vi "Menu Launch VI Information.vi"(8 "error in (no error)":errorcluster) -> (0 "error out":errorcluster, 2 "Menu Launch:VI":string, 3 "Menu Launch:App":refnum<vi>)   [LabVIEW 2020]
doc: "This VI returns the Owning Application reference and VI Name for a VI from which a Tools menu option was launched. This VI should be the first thing run on the diagram of a menu item VI."
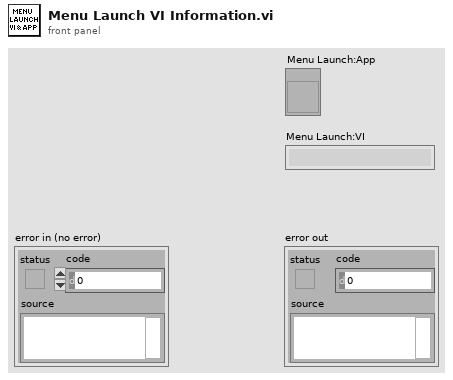
[diagram p1: front panel]
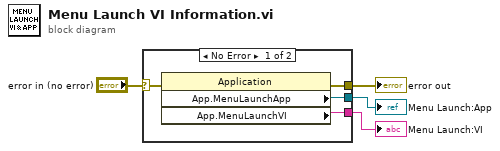
[diagram p0: block diagram]
diagram:
  n1 = case shown="No Error" "error in (no error)" {
    selector: "error in (no error)" -> [w7 w9]
    tunnel: [w8 w9] -> w4
    tunnel: [w6 _] -> w2
    tunnel: [w5 _] -> w1
    frame No Error {
      n2 = property class="Application"(error in=w7) -> (error out=w8:errorcluster, "App.MenuLaunchApp"=w6:refnum<vi>, "App.MenuLaunchVI"=w5:string)  [unwired: 1 in, 1 out]
    }
    frame Error {
    }
  }
  "error out" <- w4
  "Menu Launch:App" <- w2
  "Menu Launch:VI" <- w1
